vi "json_value.vi"(5 "text":string, 7 "ch":string, 9 "at":i32, 11 "error in (no error)":errorcluster) -> (4 "value":variant, 6 "text dup":string, 8 "ch out":string, 10 "at out":i32, 15 "error out":errorcluster)   [LabVIEW 2011]
doc: "Recursively decide what type the next value is, and return it from the correct function."
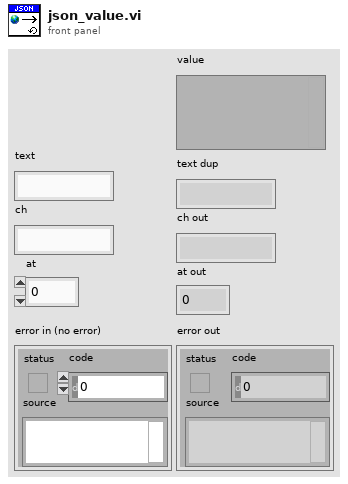
[diagram p1: front panel]
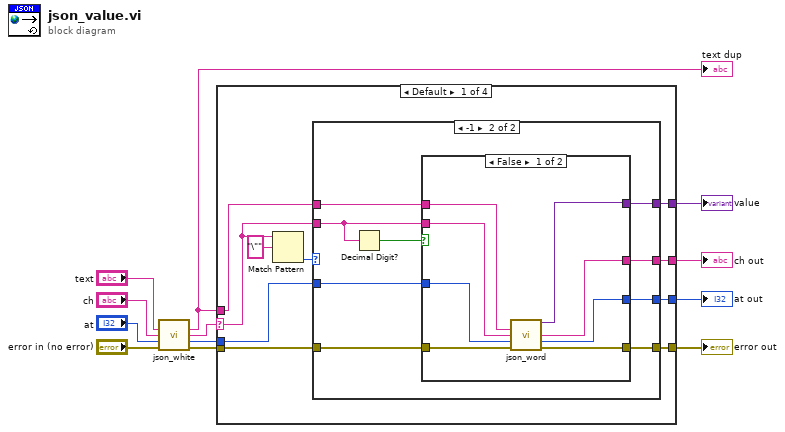
[diagram p0: block diagram]
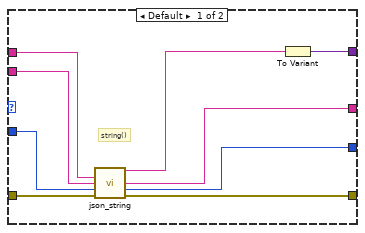
[diagram p2: hidden frame]
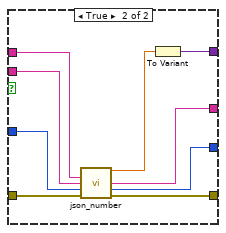
[diagram p3: hidden frame]
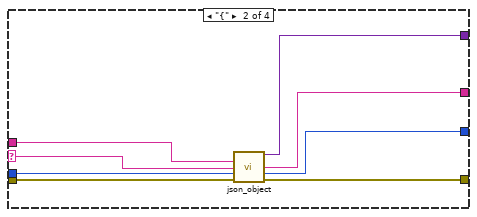
[diagram p4: hidden frame]
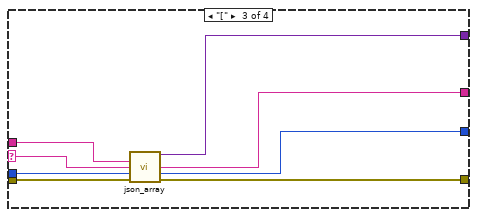
[diagram p5: hidden frame]
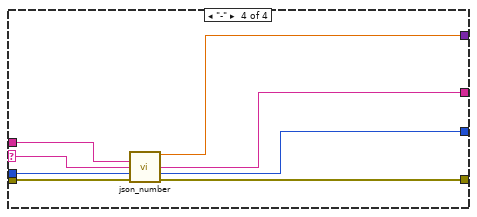
[diagram p6: hidden frame]
diagram:
  n1 = call "json_white.vi"("text"="text", "ch"="ch", "at"="at", "error in (no error)"="error in (no error)") -> ("text dup"=w5:string, "ch out"=w3:string, "at out"=w1:i32, "error out"=w7:errorcluster)  [unwired: 8 in]
  "text dup" <- w5
  n2 = case shown="Default" w3 {
    selector: w3 -> [w20 w61 w70 w78]
    tunnel: w7 -> [w19 w65 w73 w81]
    tunnel: [w18 w64 w72 w80] -> w12
    tunnel: [w17 w58 w68 w76] -> w11
    tunnel: w1 -> [w16 w63 w71 w79]
    tunnel: w5 -> [w15 w60 w69 w77]
    tunnel: [w14 w59 w67 w75] -> w10
    tunnel: [w13 w62 w66 w74] -> w9
    frame Default {
      n3 = Match Pattern(string=w20, regular expression="\"") -> (offset past match=w21:i32)  [unwired: 1 in, 3 out]
      n4 = case shown="-1" w21 {
        tunnel: w20 -> [w28 w36]
        tunnel: w19 -> [w31 w39]
        tunnel: [w30 w38] -> w18
        tunnel: [w23 w37] -> w17
        tunnel: w16 -> [w27 w35]
        tunnel: w15 -> [w29 w34]
        tunnel: [w25 w33] -> w14
        tunnel: [w26 w32] -> w13
        frame Default {
          # "string()"
          n5 = call "json_string.vi"("text"=w29, "ch"=w28, "at"=w27, "error in (no error)"=w31) -> ("string"=w24:string, "ch out"=w25:string, "at"=w26:i32, "error out"=w30:errorcluster)  [unwired: 7 in, 1 out]
          n6 = To Variant(anything=w24) -> (Variant=w23:variant)
        }
        frame -1 {
          n7 = Decimal Digit?(1:w36) -> (0:w40:bool)
          n8 = case shown="False" w40 {
            tunnel: w39 -> [w48 w57]
            tunnel: [w47 w56] -> w38
            tunnel: [w41 w49] -> w37
            tunnel: w36 -> [w45 w54]
            tunnel: w35 -> [w44 w53]
            tunnel: w34 -> [w46 w55]
            tunnel: [w42 w52] -> w33
            tunnel: [w43 w51] -> w32
            frame False {
              n9 = call "json_word.vi"("text"=w46, "ch"=w45, "at"=w44, "error in (no error)"=w48) -> ("word"=w41:variant, "ch out"=w42:string, "at out"=w43:i32, "error out"=w47:errorcluster)  [unwired: 8 in]
            }
            frame True {
              n10 = call "json_number.vi"("text"=w55, "ch"=w54, "at"=w53, "error in (no error)"=w57) -> ("number"=w50:dbl, "ch out"=w52:string, "at out"=w51:i32, "error out"=w56:errorcluster)  [unwired: 8 in]
              n11 = To Variant(anything=w50) -> (Variant=w49:variant)
            }
          }
        }
      }
    }
    frame "{" {
      n12 = call "json_object.vi"("text"=w60, "ch"=w61, "at"=w63, "error in (no error)"=w65) -> ("object"=w58:variant, "ch out"=w59:string, "at out"=w62:i32, "error out"=w64:errorcluster)  [unwired: 7 in, 1 out]
    }
    frame "[" {
      n13 = call "json_array.vi"("text"=w69, "ch"=w70, "at"=w71, "error in (no error)"=w73) -> ("array"=w68:variant, "ch out"=w67:string, "at out"=w66:i32, "error out"=w72:errorcluster)  [unwired: 7 in, 1 out]
    }
    frame "-" {
      n14 = call "json_number.vi"("text"=w77, "ch"=w78, "at"=w79, "error in (no error)"=w81) -> ("number"=w76:dbl, "ch out"=w75:string, "at out"=w74:i32, "error out"=w80:errorcluster)  [unwired: 8 in]
    }
  }
  "error out" <- w12
  "ch out" <- w10
  "at out" <- w9
  "value" <- w11
